vi "WinCI Get File Copy.vi"(6 "version":string, 8 "error in (no error)":errorcluster, 9 "target filename":path, 10 "source filename":path, 11 "source control reference in":T1) -> (0 "error out":errorcluster, 2 "status message":string, 3 "source control reference out":T1)   [LabVIEW 2020, in "NI_SCC_WinCI.lvlib"]
uses:
  <vilib>/SourceControl/Providers/WinCI/NI_SCC_WinCI.lvlib
  <vilib>/SourceControl/sccapi/SCCAPI Refnum.ctl
  <vilib>/SourceControl/sccapi/SCCAPI Get Retrieval Method.ctl
  <vilib>/SourceControl/support/SCCSup Message Strings GLBL.vi
  <vilib>/SourceControl/sccapi/NI_SCC.lvlib
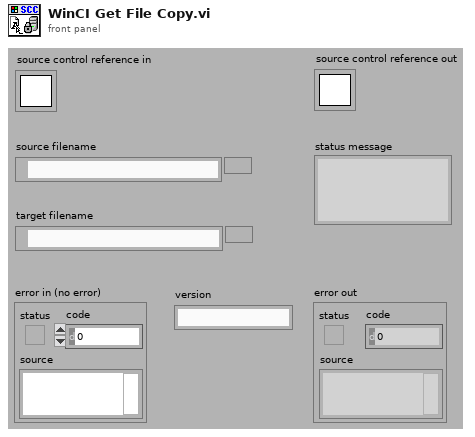
[diagram p1: front panel]
types:
  T1 = typedef "NI_SCC.lvlib/SCCAPI Refnum.ctl" = refnum<k1>
  T2 = typedef "NI_SCC.lvlib/SCCAPI SCC File Status.ctl" = cluster{"in source control?":bool, "checked out by user?":bool, "checked out by other?":bool, "out of date?":bool, "deleted?":bool}
  T3 = typedef "NI_SCC.lvlib/SCCAPI Get Retrieval Method.ctl" = u16
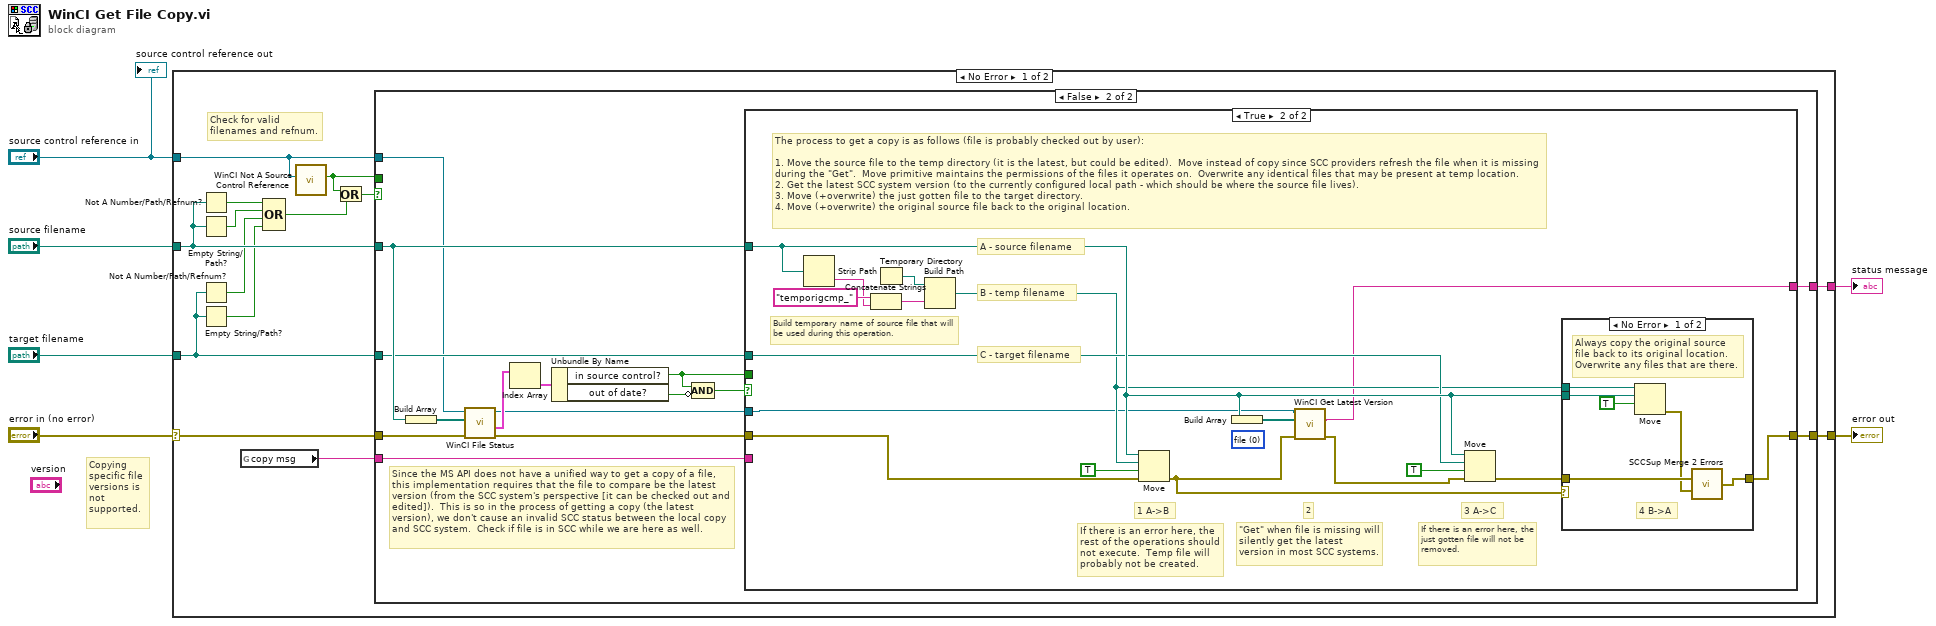
[diagram p0: block diagram]
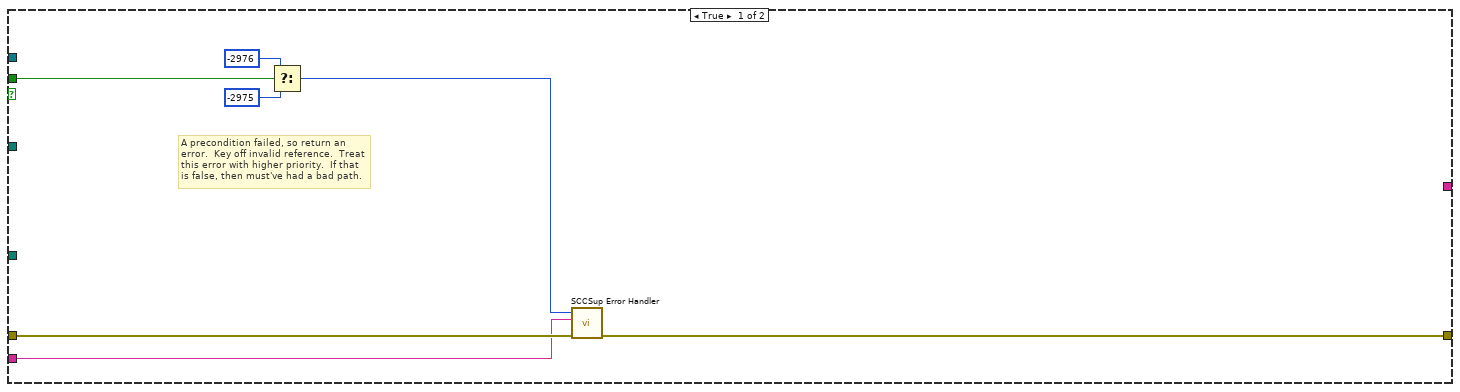
[diagram p2: hidden frame]
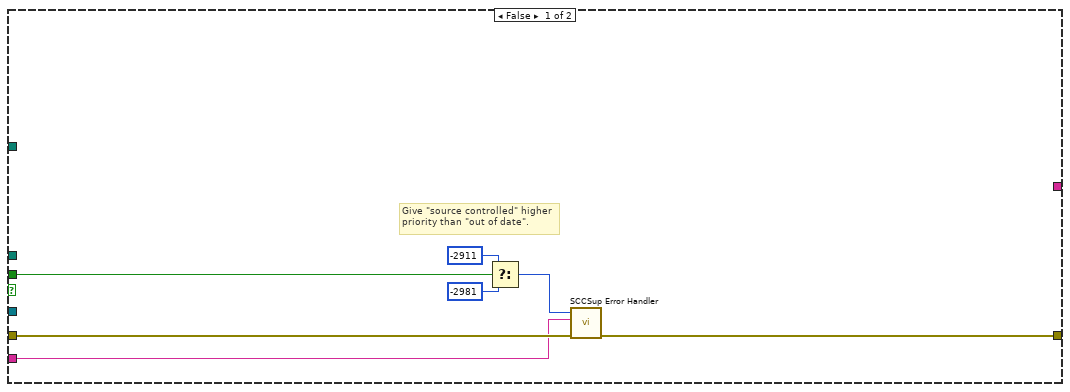
[diagram p3: hidden frame]
diagram:
  # "Copying specific file versions is not supported."
  n1 = case shown="No Error" "error in (no error)" {
    selector: "error in (no error)" -> [w11 w74]
    tunnel: [w10 w74] -> w5
    tunnel: "source control reference in" -> [w7 _]
    tunnel: [w20 _] -> w3
    tunnel: "source filename" -> [w16 _]
    tunnel: "target filename" -> [w14 _]
    frame No Error {
      # "Check for valid filenames and refnum."
      n2 = Not A Number/Path/Refnum?(number/path/refnum=w16) -> (NaN/Path/Refnum?=w17:bool)
      n3 = Empty String/Path?(string/path=w16) -> (empty?=w18:bool)
      n4 = Not A Number/Path/Refnum?(number/path/refnum=w14) -> (NaN/Path/Refnum?=w13:bool)
      n5 = Empty String/Path?(string/path=w14) -> (empty?=w12:bool)
      n6 = global read "SCCSup Message Strings GLBL.vi" "copy msg"() -> (w9:string)
      n7 = Compound Arithmetic op=OR(w17, w18, w13, w12) -> (w19:bool)
      n8 = call <vilib>:"WinCI Not A Source Control Reference.vi"("source control reference in"=w7) -> ("not a source control reference?"=w8:bool)  [unwired: 1 in, 9 out]
      n9 = Or(x=w8, y=w19) -> (x .or. y?=w15:bool)
      n10 = case shown="False" w15 {
        tunnel: w7 -> [_ w28]
        tunnel: [_ w37] -> w20
        tunnel: w16 -> [_ w35]
        tunnel: w14 -> [_ w34]
        tunnel: w8 -> [w25 _]
        tunnel: w11 -> [w24 w32]
        tunnel: [w22 w38] -> w10
        tunnel: w9 -> [w21 w36]
        frame True {
          # "A precondition failed, so return an error.  Key off invalid reference.  Treat this error with higher priority.  If that is false, then must've had a bad path."
          n11 = Select(t=-2976 ("result"), s=w25, f=-2975 ("result")) -> (s? t:f=w23:i32)
          n12 = call <vilib>:"SCCSup Error Handler.vi"("error in (no error)"=w24, "operation message"=w21, "scc error code"=w23) -> ("error out"=w22:errorcluster)  [unwired: 1 in, 7 out]
        }
        frame False {
          # "Since the MS API does not have a unified way to get a copy of a file, this implementation requires that the file to compare be the latest version (from the SCC system's perspective [it can be checked out and edited]).  This is so in the process of getting a copy (the latest version), we don't cause an invalid SCC status between the local copy and SCC system.  Check if file is in SCC while we are here as well."
          n13 = Build Array(w35) -> (w33:path[])
          n14 = call <vilib>:"WinCI File Status.vi"("error in (no error)"=w32, "files"=w33, "source control reference in"=w28) -> ("error out"=w31:errorcluster, "file status"=w30:T2[], "source control reference out"=w29:T1)  [unwired: 6 out]
          n15 = Index Array(array=w30) -> (element=w42:T2)  [unwired: 1 in]
          n16 = Unbundle By Name(w42) -> ("in source control?"=w39:bool, "out of date?"=w40:bool)
          n17 = Compound Arithmetic op=AND(w39, invert w40) -> (w41:bool)
          n18 = case shown="True" w41 {
            tunnel: w31 -> [w49 w62]
            tunnel: w29 -> [_ w52]
            tunnel: [w48 w57] -> w38
            tunnel: w39 -> [w44 _]
            tunnel: [_ w53] -> w37
            tunnel: w36 -> [w43 _]
            tunnel: w35 -> [_ w59]
            tunnel: w34 -> [_ w56]
            frame False {
              # "Give \"source controlled\" higher priority than \"out of date\"."
              n19 = Select(t=-2911 ("error code"), s=w44, f=-2981) -> (s? t:f=w47:i32)
              n20 = call <vilib>:"SCCSup Error Handler.vi"("error in (no error)"=w49, "operation message"=w43, "scc error code"=w47) -> ("error out"=w48:errorcluster)  [unwired: 1 in, 7 out]
            }
            frame True {
              (unwired) T3 0 items=["file", "directory", "directory (recursive)"] ("retrieval method (file)")
              # "If there is an error here, the just gotten file will not be removed."
              # "\"Get\" when file is missing will silently get the latest version in most SCC systems."
              # "If there is an error here, the rest of the operations should not execute.  Temp file will probably not be created."
              # "B - temp filename"
              # "C - target filename"
              # "A - source filename"
              # "Build temporary name of source file that will be used during this operation."
              # "3 A->C"
              # "2"
              # "1 A->B"
              # "The process to get a copy is as follows (file is probably checked out by user):\n\n1. Move the source file to the temp directory (it is the latest, but could be edited).  Move instead of copy since SCC providers refresh the file when it is missing during the \"Get\".  Move primitive maintains the permissions of the files it operates on.  Overwrite any identical files that may be present at temp location.\n2. Get the latest SCC system version (to the currently configured local path - which should be where the source file lives).\n3. Move (+overwrite) the just gotten file to the target directory.\n4. Move (+overwrite) the original source file back to the original location."
              n21 = Strip Path(path=w59) -> (name=w64:string)  [unwired: 1 out]
              n22 = Concatenate Strings("temporigcmp_" ("name or relative path"), w64) -> (w63:string)
              n23 = Temporary Directory() -> (w65:path)
              n24 = Build Path(base path=w65, name or relative path=w63) -> (appended path=w55:path)
              n25 = Move(source path=w59, error in=w62, 9:TRUE ("overwrite (F)"), 10:w55) -> (error out=w51:errorcluster)  [unwired: 3 out]
              n26 = Build Array(w59) -> (w54:path[])
              n27 = call <vilib>:"WinCI Get Latest Version.vi"("error in (no error)"=w51, "files"=w54, "source control reference in"=w52) -> ("error out"=w50:errorcluster, "status message"=w53:string)  [unwired: 1 in, 6 out]
              n28 = Move(source path=w59, error in=w50, 9:TRUE ("overwrite (F)"), 10:w56) -> (error out=w58:errorcluster)  [unwired: 3 out]
              n29 = case shown="No Error" w51 {
                tunnel: w55 -> [w72 _]
                tunnel: w59 -> [w70 _]
                tunnel: w58 -> [w69 w73]
                tunnel: [w67 w73] -> w57
                frame No Error {
                  # "Always copy the original source file back to its original location.  Overwrite any files that are there."
                  # "4 B->A"
                  n30 = Move(source path=w72, 9:TRUE ("overwrite (F)"), 10:w70) -> (error out=w68:errorcluster)  [unwired: 1 in, 3 out]
                  n31 = call <vilib>:"SCCSup Merge 2 Errors.vi"("Error IO 1"=w69, "Error IO 2"=w68) -> ("Error IO out"=w67:errorcluster)  [unwired: 13 out]
                }
                frame Error {
                  # "Don't try to move temp file back since it was never moved due to an error."
                }
              }
            }
          }
        }
      }
    }
    frame Error {
    }
  }
  "error out" <- w5
  "status message" <- w3
  "source control reference out" <- "source control reference in"
